vi "S2DS_EditWCReadFromFileInfo.vi"(11 "WC read from file info (out) in":T1) -> (2 "Sweep continue":bool, 3 "WC read from file info (out) out":T1)   [LabVIEW 2025]
uses:
  TYPE DEFS/S2DS_WCFromFileInfo.ctl
  <vilib>/Utility/file.llb/Read Delimited Spreadsheet (string).vi
  <vilib>/Utility/file.llb/Read Delimited Spreadsheet (DBL).vi
panel:
  out "Column":i32
  out "String":string
  in  "Reload":bool
  out "Total\nline":i32
  in  "CANCEL":bool
  in  "OK":bool
  in  "Starting\nrow":u32=1 min=1
  in  "File Path from where to read WC targets":path
  # "CHOOSE FILE & LINE NO \nfor targets of WC..."
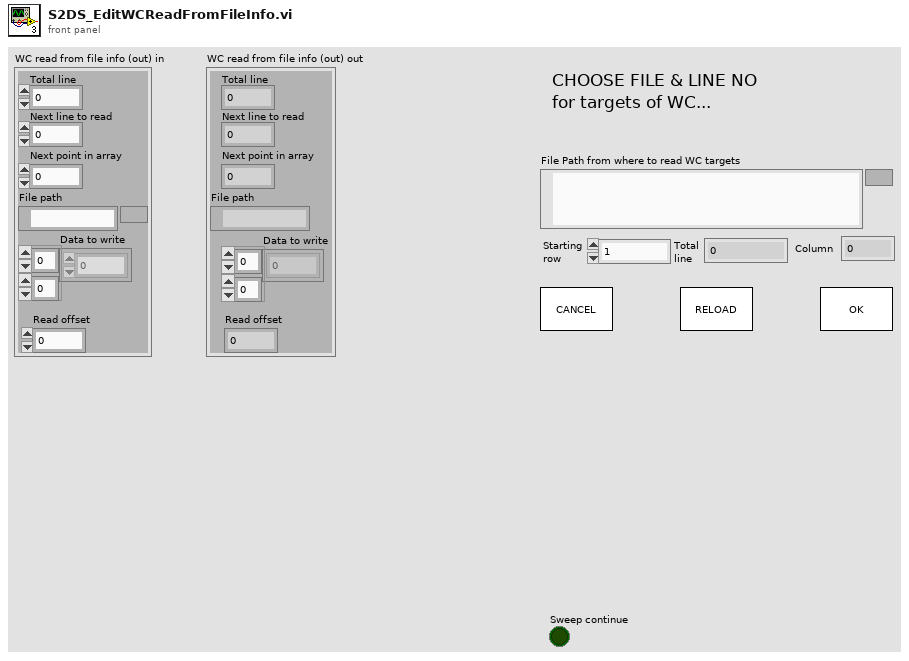
[diagram p1: front panel]
types:
  T1 = typedef "S2DS_WCFromFileInfo.ctl" = cluster{"Next line to read":i32, "Next point in array":i32, "File path":path, "Data to write":dbl[][], "Read offset":i32, "Total line":i32}
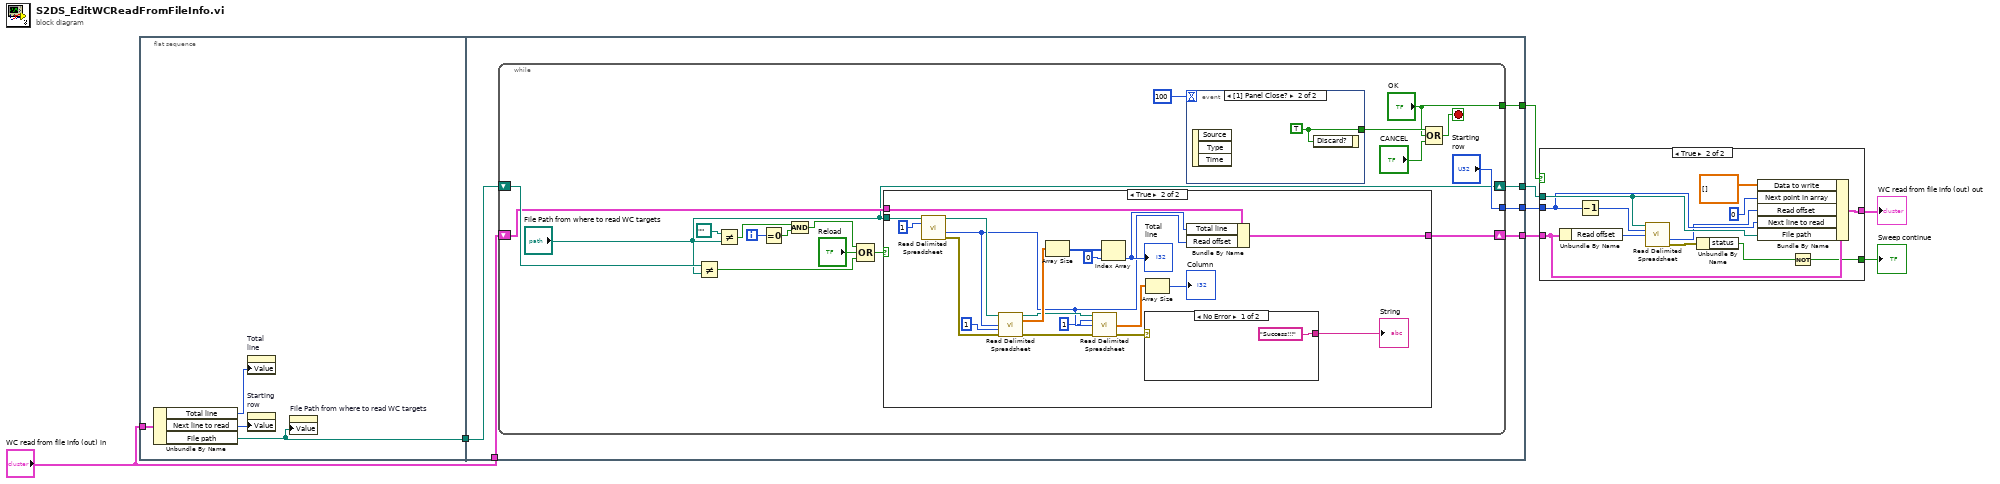
[diagram p0: block diagram]
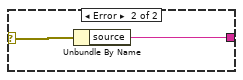
[diagram p4: hidden frame]
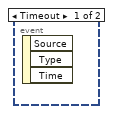
[diagram p5: hidden frame]
diagram:
  n1 = flat-sequence {
    tunnel: "WC read from file info (out) in" -> [w12]
    tunnel: [w11] -> w4
    tunnel: [w18] -> w6
    tunnel: [w16] -> w5
    tunnel: [w17] -> w8
    tunnel: w4 -> [w15]
    tunnel: "WC read from file info (out) in" -> [w14]
    tunnel: [w13] -> w2
    frame #0 {
      n2 = Unbundle By Name(w12) -> ("Total line"=w9:i32, "Next line to read"=w10:i32, "File path"=w11:path)
      n3 = property on="Total\nline" class="DigNum (strict)"("Value"=w9) -> ()  [unwired: 2 in, 2 out]
      n4 = property on="Starting\nrow" class="DigNum (strict)"("Value"=w10) -> ()  [unwired: 2 in, 2 out]
      n5 = property on="File Path from where to read WC targets" class="Path"("Value"=w11) -> ()  [unwired: 2 in, 2 out]
    }
    frame #1 {
      n6 = while {
        tunnel: ["Starting\nrow"] -> w18
        tunnel: ["OK"] -> w17
        shift-right: ["File Path from where to read WC targets"] -> w16
        shift-left: w15 -> [w30]
        shift-right: [w29] -> w13
        shift-left: w14 -> [w28]
        i -> [w24]
        stop <- w34 stop-if-true
        n7 = Not Equal?(x=w30, y="File Path from where to read WC targets") -> (x != y?=w26:bool)
        n8 = Not Equal?(x=path "", y="File Path from where to read WC targets") -> (x != y?=w21:bool)
        n9 = Equal To 0?(x=w24) -> (x = 0?=w20:bool)
        n10 = And(x=w21, y=w20) -> (x .and. y?=w19:bool)
        n11 = Compound Arithmetic op=OR(w19, "Reload", w26) -> (w25:bool)
        n12 = case shown="True" w25 {
          tunnel: [w37 w53] -> w29
          tunnel: w28 -> [w37 w54]
          tunnel: "File Path from where to read WC targets" -> [_ w55]
          frame False {
          }
          frame True {
            n13 = call-poly <vilib>:"Read Delimited Spreadsheet.vi"("file path (dialog if empty)"=w55, "number of rows (all:-1)"=1) -> ("new file path (Not A Path if cancelled)"=w52:path, "mark after read (chars.)"=w41:i32, "error out"=w51:errorcluster)  [unwired: 8 in, 3 out]
            n14 = call-poly <vilib>:"Read Delimited Spreadsheet.vi"("file path (dialog if empty)"=w52, "start of read offset (chars.:0)"=w41, "max characters/row  (no limit:0)"=1, "error in (no error)"=w51) -> ("new file path (Not A Path if cancelled)"=w44:path, "all rows"=w49:dbl[][], "error out"=w43:errorcluster)  [unwired: 6 in, 3 out]
            n15 = Array Size(array=w49) -> (size(s)=w48:i32[])
            n16 = call-poly <vilib>:"Read Delimited Spreadsheet.vi"("file path (dialog if empty)"=w44, "number of rows (all:-1)"=1, "start of read offset (chars.:0)"=w41, "error in (no error)"=w43) -> ("first row"=w39:dbl[], "error out"=w42:errorcluster)  [unwired: 6 in, 4 out]
            n17 = Index Array(array=w48, index=0) -> (element=w46:i32)
            "Total\nline" <- w46
            n18 = case shown="No Error" w42 {
              selector: w42 -> [_ w59]
              tunnel: ["Success!!!" w58] -> w45
              frame No Error {
              }
              frame Error {
                n19 = Unbundle By Name(w59) -> ("source"=w58:string)
              }
            }
            "String" <- w45
            n20 = Array Size(array=w39) -> (size(s)=→"Column":i32)
            n21 = Bundle By Name(cluster=w54, "Total line"=w46, "Read offset"=w41) -> (w53:T1)
          }
        }
        n22 = event shown="[1] Panel Close?" {
          selector: _ -> [_ _]
          dyn-events: _ -> [_ _]
          timeout: 100 -> [_ _]
          tunnel: [_ w60] -> w35
          event Timeout {
            n23 = event-data() -> ()  [unwired: 1 in, 3 out]
          }
          event Panel Close? {
            w60 = TRUE ("Discard?")
            n24 = event-data() -> ()  [unwired: 1 in, 3 out]
            n25 = event-data("Discard?"=w60) -> ()  [unwired: 1 in, 1 out]
          }
        }
        n26 = Compound Arithmetic op=OR(w35, "OK", "CANCEL") -> (w34:bool)
      }
    }
  }
  n27 = case shown="True" w8 {
    selector: w8 -> [w61 _]
    tunnel: [w62 w74] -> w7
    tunnel: w2 -> [w62 w68]
    tunnel: w6 -> [_ w72]
    tunnel: w5 -> [_ w73]
    tunnel: [w61 w63] -> w1
    frame False {
    }
    frame True {
      n28 = Unbundle By Name(w68) -> ("Read offset"=w67:i32)
      n29 = Decrement(x=w72) -> (x-1=w71:u32)
      n30 = call-poly <vilib>:"Read Delimited Spreadsheet.vi"("file path (dialog if empty)"=w73, "number of rows (all:-1)"=w71, "start of read offset (chars.:0)"=w67) -> ("mark after read (chars.)"=w70:i32, "error out"=w65:errorcluster)  [unwired: 7 in, 4 out]
      n31 = Unbundle By Name(w65) -> ("status"=w64:bool)
      n32 = Bundle By Name(cluster=w68, "Data to write"=dbl[][] [], "Next point in array"=0 ("Current index"), "Read offset"=w70, "Next line to read"=w72, "File path"=w73) -> (w74:T1)
      n33 = Not(x=w64) -> (.not. x?=w63:bool)
    }
  }
  "WC read from file info (out) out" <- w7
  "Sweep continue" <- w1
